vi "SetAttributeViReal64_SA-Limit_Mask.vi"(7 "AttributeValue":dbl, 8 "error in (no error)":errorcluster {"code" format="%.0x"}, 9 "AttributeID":u32(ring)=1150624 items=["SA_LIMIT_MARGIN"=1150624, "SA_LIMIT_X_OFFSET"=1150631, "SA_LIMIT_Y_OFFSET"=1150632, "SA_SEMASK_DISPLAY_WINDOWX_REFERENCE"=1150814, "SA_SEMASK_DISPLAY_WINDOWX_SCALE"=1150815, "SA_SEMASK_DISPLAY_WINDOWY_REFERENCE"=1150385, "SA_SEMASK_DISPLAY_WINDOWY_SCALE"=1150388, "SA_SEMASK_MARKER_POSITION"=1150406, "SA_SEMASK_OFFSETFILTER_ALPHA"=1150381, "SA_SEMASK_REFERENCECHANNEL_CPSD"=1150362, "SA_SEMASK_REFERENCECHANNEL_FREQUENCY_SPAN"=1150368, "SA_SEMASK_REFERENCECHANNEL_PEAK_POWER"=1150365, "SA_SEMASK_REFERENCECHANNEL_TOTAL_POWER"=1150363, "SA_SEMASK_SWEEPCOUPLING_BANDWIDTH_RATIO"=1150374, "SA_SEMASK_SWEEPCOUPLING_CHANNEL_INTEGRATION_BANDWIDTH"=1150371, "SA_SEMASK_SWEEPCOUPLING_RESOLUTION_BANDWIDTH"=1150372, "SA_SEMASK_SWEEPCOUPLING_SWEEP_TIME"=1150375, "SA_SEMASK_SWEEPCOUPLING_VIDEO_BANDWIDTH"=1150378], 10 "RepCapIdentifier":string, 11 "instrument handle":refnum<k15>) -> (0 "error out":errorcluster {"code" format="%.0x"}, 3 "instrument handle out":refnum<k15>)   [LabVIEW 2009, in "Keysight XSAn.lvlib"]
doc: "Sets a Real64 attribute from the instrument driver.\nThe following Attributes are supported:\n\nSA_LIMIT_MARGIN\nSA_LIMIT_X_OFFSET\nSA_LIMIT_Y_OFFSET\nSA_SEMASK_DISPLAY_WINDOWX_REFERENCE\nSA_SEMASK_DISPLAY_WINDOWX_SCALE\nSA_SEMASK_DISPLAY_WINDOWY_REFERENCE\nSA_SEMASK_DISPLAY_WINDOWY_SCALE\nSA_SEMASK_MARKER_POSITION\nSA_SEMASK_OFFSETFILTER_ALPHA\nSA_SEMASK_REFERENCECHANNEL_CPSD\nSA_SEMASK_REFERENCECHANNEL_FREQUENCY_SPAN\nSA_SEMASK_REFERENCECHANNEL_PEAK_POWER\nSA_SEMASK_REFERENCECHANNEL_TOTAL_POWER\nSA_SEMASK_SWEEPCOUPLING_BANDWIDTH_RATIO\nSA_SEMASK_SWEEPCOUPLING_CHANNEL_INTEGRATION_BANDWIDTH\nSA_SEMASK_SWEEPCOUPLING_RESOLUTION_BANDWIDTH\nSA_SEMASK_SWEEPCOUPLING_SWEEP_TIME\nSA_SEMASK_SWEEPCOUPLING_VIDEO_BANDWIDTH"
uses:
  <instrlib>/Keysight XSAn/Keysight XSAn.lvlib
  AgXSAn.dll
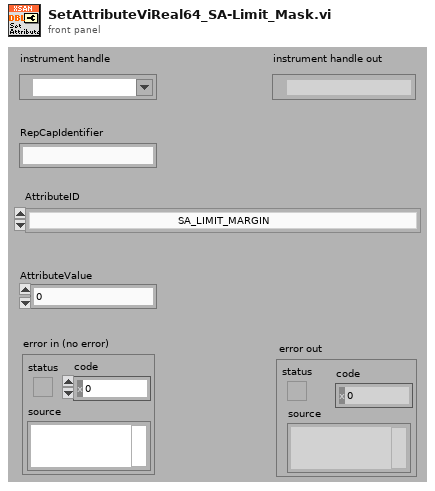
[diagram p1: front panel]
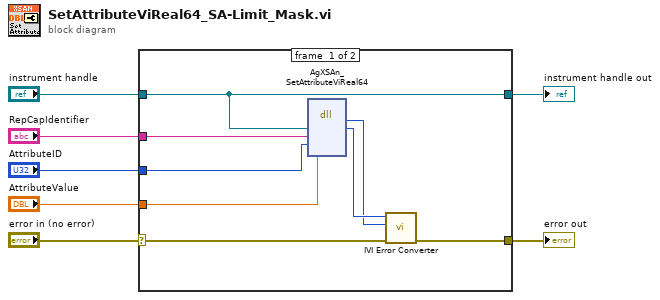
[diagram p0: block diagram]
diagram:
  n1 = case shown="No Error" "error in (no error)" {
    selector: "error in (no error)" -> [w13 w17]
    tunnel: [w12 w17] -> w7
    tunnel: "instrument handle" -> [w8 w16]
    tunnel: "RepCapIdentifier" -> [w11 _]
    tunnel: "AttributeID" -> [w10 _]
    tunnel: "AttributeValue" -> [w9 _]
    tunnel: [w8 w16] -> w1
    frame #0 {
      n2 = dll-call lib="AgXSAn**.dll" fn="AgXSAn_SetAttributeViReal64"("Vi"=w8, "RepCapIdentifier"=w11, "AttributeID"=w10, "AttributeValue"=w9) -> ("return type"=w14:i32, "Vi"=w15:u32)  [unwired: 6 in, 2 out]
      n3 = call <instrlib>:"IVI Error Converter.vi"("error in (no error)"=w13, "IVI error code (0)"=w14, "instrument handle"=w15) -> ("error out"=w12:errorcluster)  [unwired: 7 in, 1 out]
    }
    frame #1 {
    }
  }
  "error out" <- w7
  "instrument handle out" <- w1
